vi "Validate Table Column Name.vi"(8 "error in":errorcluster, 11 "Table Display Name in":string) -> (0 "error out":errorcluster, 3 "Table Display Name out":string)   [LabVIEW 2019, in "Open Xml.lvlib"]
uses:
  Open Xml.lvlib
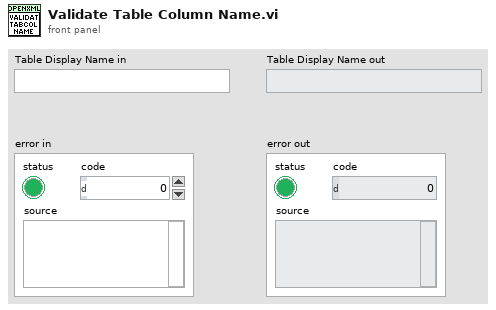
[diagram p1: front panel]
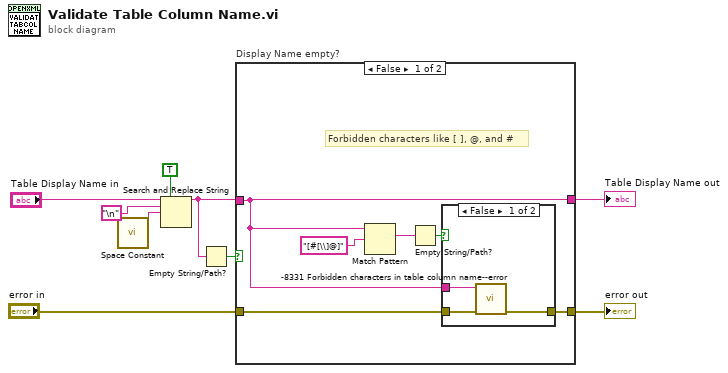
[diagram p0: block diagram]
diagram:
  n1 = call <vilib>:"Space Constant.vi"() -> ("String"=w3:string)
  n2 = Search and Replace String(replace all?=TRUE ("replace all? (F)"), input string="Table Display Name in", search string="\n", replace string=w3) -> (result string=w1:string)  [unwired: 4 in, 3 out]
  n3 = Empty String/Path?(string/path=w1) -> (empty?=w7:bool)
  n4 = case "Display Name empty?" shown="False" w7 {
    tunnel: "error in" -> [w15 w20]
    tunnel: [w14 w20] -> w8
    tunnel: w1 -> [w10 w21]
    tunnel: [w10 w21] -> w6
    frame False {
      # "Forbidden characters like [ ], @, and #"
      n5 = Match Pattern(string=w10, regular expression="[#[\\]@]") -> (match substring=w12:string)  [unwired: 1 in, 3 out]
      n6 = Empty String/Path?(string/path=w12) -> (empty?=w11:bool)
      n7 = case shown="False" w11 {
        tunnel: w15 -> [w18 w19]
        tunnel: [w17 w19] -> w14
        tunnel: w10 -> [w16 _]
        frame False {
          n8 = call "-8331 Forbidden characters in table column name--error.vi"("error in"=w18, "Argument"=w16) -> ("error out"=w17:errorcluster)  [unwired: 8 in, 1 out]
        }
        frame True {
        }
      }
    }
    frame True {
    }
  }
  "error out" <- w8
  "Table Display Name out" <- w6
